vi "clusters.vi"() -> ()   [LabVIEW 2020]
panel:
  out "Ubidots_HTTP.Device Label":string
  out "Data_PLC.Direccion IP":string
  out "Data_Microcontrolador.ADC":dbl[](array[numeric])
  out "Cluster Industrial":T1
  in  "Numeric":u16
  in  "Trama JSON":string
  in  "Salidas PLC S71200":bool[](array[boolean])
  in  "Termocupla 1":dbl(slide) scale=0.0..100.0
  in  "Variador de Velocidad 2":dbl
  out "Cluster Indicador de Pesadora":T2
  out "Variador de Velocidad":dbl
  out "Monitor Remoto":string
  out "START":bool
  in  "Pesadora Automatica":T2 {"Variador de Velocidad" scale=0.0..60.0}
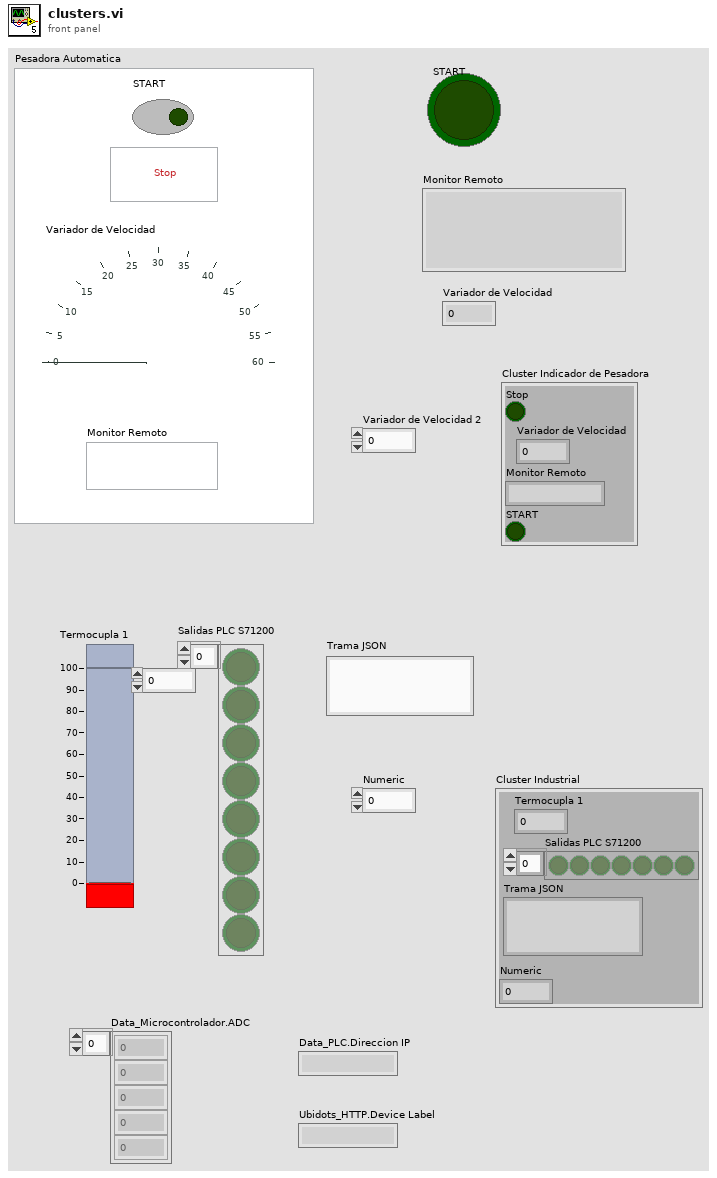
[diagram p1: front panel]
types:
  T1 = cluster{"Termocupla 1":dbl, "Salidas PLC S71200":bool[], "Trama JSON":string, "Numeric":u16}
  T2 = cluster{"Stop":bool, "Variador de Velocidad":dbl, "Monitor Remoto":string, "START":bool}
  T3 = cluster{"Data_Microcontrolador":cluster{"ADC":dbl[], "ON/OFF":bool, "Mensaje Uart":string}, "Data_PLC":cluster{"Direccion IP":string, "Puerto":i32, "Pinzadora":i32[], "V_Variadores":dbl[]}, "Ubidots_HTTP":cluster{"Dominio":string, "Puerto TCP":i32, "Token":string, "Device Label":string, "Formato JSON":string, "Temp_casa":dbl}}
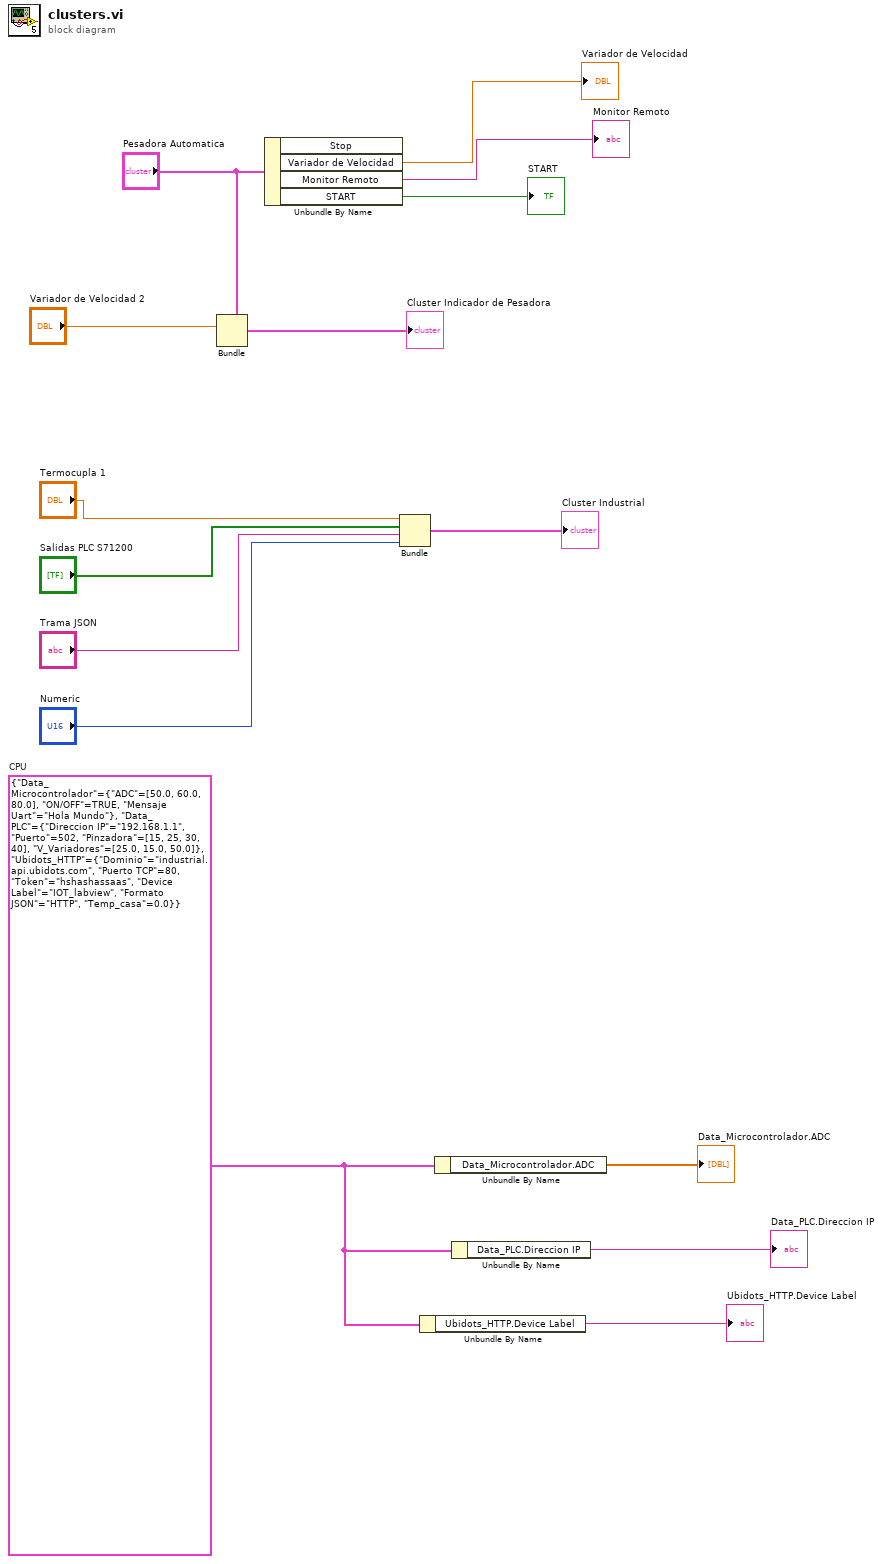
[diagram p0: block diagram]
diagram:
  w4 = T3 {"Data_Microcontrolador"={"ADC"=[50.0, 60.0, 80.0], "ON/OFF"=TRUE, "Mensaje Uart"="Hola Mundo"}, "Data_PLC"={"Direccion IP"="192.168.1.1", "Puerto"=502, "Pinzadora"=[15, 25, 30, 40], "V_Variadores"=[25.0, 15.0, 50.0]}, "Ubidots_HTTP"={"Dominio"="industrial.api.ubidots.com", "Puerto TCP"=80, "Token"="hshashassaas", "Device Label"="IOT_labview", "Formato JSON"="HTTP", "Temp_casa"=0.0}}  # CPU
  n1 = Bundle(cluster="Pesadora Automatica", "Variador de Velocidad"="Variador de Velocidad 2") -> (→"Cluster Indicador de Pesadora":T2)  [unwired: 3 in]
  n2 = Unbundle By Name("Pesadora Automatica") -> ("Variador de Velocidad"=→"Variador de Velocidad":dbl, "Monitor Remoto"=→"Monitor Remoto":string, "START"=→"START":bool)  [unwired: 1 out]
  n3 = Bundle("Termocupla 1"="Termocupla 1", "Salidas PLC S71200"="Salidas PLC S71200", "Trama JSON"="Trama JSON", "Numeric"="Numeric") -> (→"Cluster Industrial":T1)  [unwired: 1 in]
  n4 = Unbundle By Name(w4) -> ("Ubidots_HTTP.Device Label"=→"Ubidots_HTTP.Device Label":string)
  n5 = Unbundle By Name(w4) -> ("Data_Microcontrolador.ADC"=→"Data_Microcontrolador.ADC":dbl[])
  n6 = Unbundle By Name(w4) -> ("Data_PLC.Direccion IP"=→"Data_PLC.Direccion IP":string)
